vi "Get Async Buffer.vi"(11 "Buffers in":refnum<class "Buffers.lvclass">) -> (2 "Async Buffer":refnum<class "Buffer.lvclass">, 3 "Buffers out":refnum<class "Buffers.lvclass">)   [LabVIEW 2017, in "DSF Core.lvlib" / "Buffers.lvclass"]
uses:
  Buffers.lvclass
  Buffer.lvclass
  Buffers.lvclass/Buffers.ctl
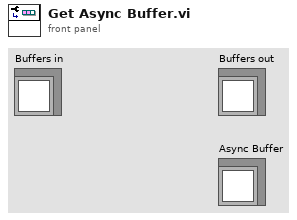
[diagram p1: front panel]
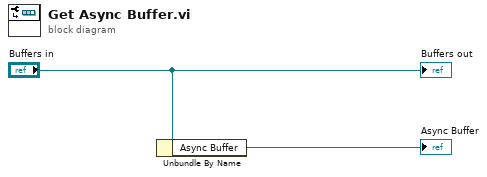
[diagram p0: block diagram]
diagram:
  n1 = Unbundle By Name("Buffers in") -> ("Async Buffer"=→"Async Buffer":refnum<class "Buffer.lvclass">)
  "Buffers out" <- "Buffers in"
